vi "CoordinateTransformMatrix_To_Transform.vi"(3 "Linear conversion Matrix":dbl[][](array[numeric])) -> (1 "Transform (Center first)":T1)   [LabVIEW 2011]
panel:
  out "c":dbl
  out "invers Conversion Matrix":dbl[][](array[numeric])
  # "unterbestimmt nur für rechtwinklig: |a|=|c| und |b|=|c|\nmirror: tauscht bei b,d vorzeichen"
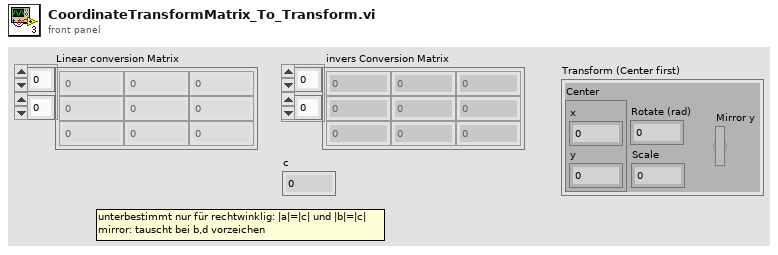
[diagram p1: front panel]
types:
  T1 = cluster{"Center":cluster{"x":dbl, "y":dbl}, "Rotate (rad)":dbl, "Mirror y":bool, "Scale":dbl}
  T2 = cluster{" invers Conversion Matrix[0]":dbl, " invers Conversion Matrix[1]":dbl}
  T3 = cluster{" invers Conversion Matrix":cluster{" invers Conversion Matrix[0]":dbl, " invers Conversion Matrix[1]":dbl}, "w":dbl, bool, "s":dbl}
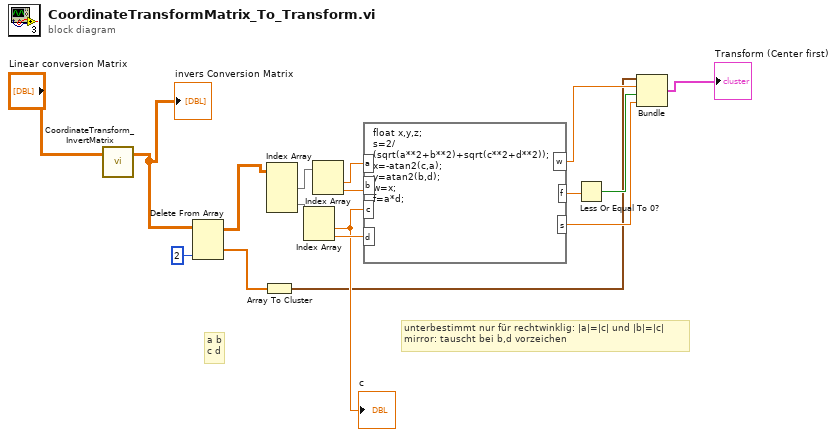
[diagram p0: block diagram]
diagram:
  # "a b\nc d"
  # "unterbestimmt nur für rechtwinklig: |a|=|c| und |b|=|c|\nmirror: tauscht bei b,d vorzeichen"
  n1 = call "CoordinateTransform_InvertMatrix.vi"("Conversion Matrix"="Linear conversion Matrix") -> ("invers Conversion Matrix"=w2:dbl[][])  [unwired: 1 in, 1 out]
  "invers Conversion Matrix" <- w2
  n2 = Delete From Array(array=w2, index (col)=2 ("disabled index (col)")) -> (deleted portion=w4:dbl[], array with subset deleted=w7:dbl[][])  [unwired: 2 in]
  n3 = Array To Cluster(array=w4) -> (cluster=w6:T2)
  n4 = Index Array(array=w7) -> (element #1=w8:dbl[], element #2=w9:dbl[])  [unwired: 4 in]
  n5 = Index Array(array=w9) -> (element #1=w12:dbl, element #2=w13:dbl)  [unwired: 2 in]
  "c" <- w12
  n6 = Index Array(array=w8) -> (element #1=w10:dbl, element #2=w11:dbl)  [unwired: 2 in]
  n7 = formula code="float x,y,z;\ns=2/(sqrt(a**2+b**2)+sqrt(c**2+d**2));\nx=-atan2(c,a);\ny=atan2(b,d);\nw=x;\nf=a*d;"("a"=w10, "b"=w11, "c"=w12, "d"=w13) -> ("w"=w14:dbl, "s"=w15:dbl, "f"=w16:dbl)
  n8 = Less Or Equal To 0?(x=w16) -> (x <= 0?=w17:bool)
  n9 = Bundle("invers Conversion Matrix"=w6, "w"=w14, w17, "s"=w15) -> (→"Transform (Center first)":T3)  [unwired: 1 in]
